vi "QT_QTImageToLVPict.vi"(1 "Draw info":bool, 2 "Image/Movie Out":T1={"Width"=160, "Height"=120, "Depth"=32, "data"=[], "Compressed data"=[], "Color table"=[], "Duration"=0, "Options"=0, "Timestamp"=0, "ID"=616, "Reserved"=0, "Dialogs"=0} {"Dialogs" format="%.0b"}, 3 "BW image":bool) -> (9 "Timestamp":i32, 13 "ID":i32=616, 14 "Picture color":picture, 16 "Picture B&W/Alpha channel":picture, 19 "Pict Draw Area Size":cluster{"Width":i16, "Height":i16}={"Width"=160, "Height"=120})   [LabVIEW 2024]
uses:
  <userlib>/ImageProcessing/QTLIB_2595_LV86/QT_Image.ctl
panel:
  in  "1 bit image":bool
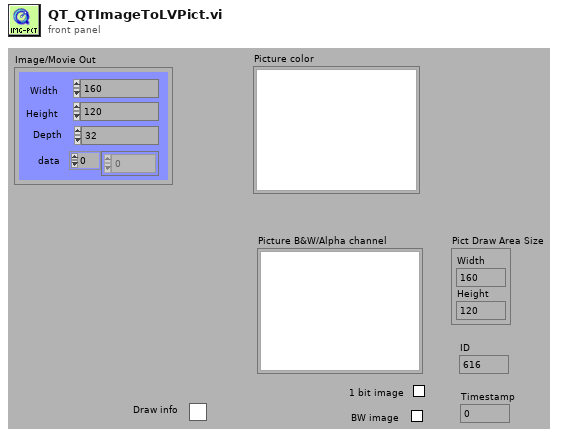
[diagram p1: front panel]
types:
  T1 = typedef "QT_Image.ctl" = cluster{"Width":i32, "Height":i32, "Depth":i32, "data":u8[], "Compressed data":u8[], "Color table":u32[], "Duration":i32, "Options":i32, "Timestamp":i32, "ID":i32, "Reserved":i32, "Dialogs":u32}
  T2 = cluster{"left":i16, "top":i16, "right":i16, "bottom":i16}
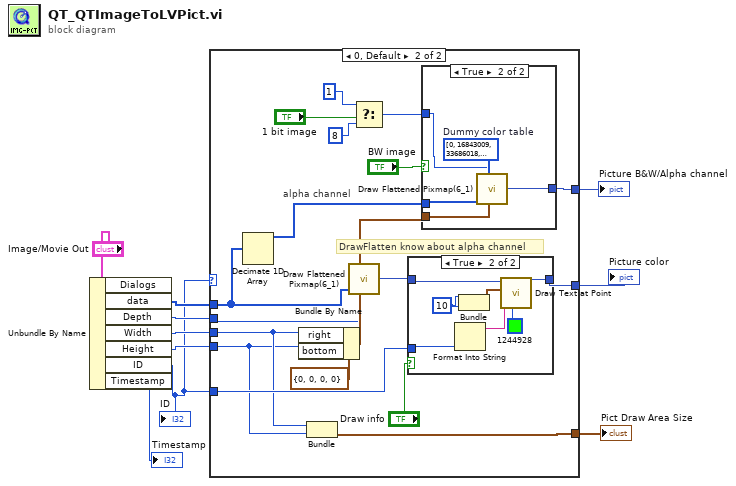
[diagram p0: block diagram]
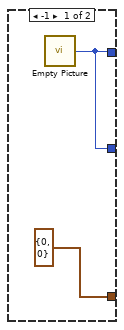
[diagram p2: hidden frame]
diagram:
  n1 = Unbundle By Name("Image/Movie Out") -> ("data"=w10:u8[], "Depth"=w8:i32, "Width"=w7:i32, "Height"=w6:i32, "ID"=w3:i32, "Timestamp"=→"Timestamp":i32)  [unwired: 1 out]
  "ID" <- w3
  n2 = case shown="0, Default" w3 {
    tunnel: w10 -> [_ w13]
    tunnel: w8 -> [_ w19]
    tunnel: w7 -> [_ w21]
    tunnel: w6 -> [_ w20]
    tunnel: [w12 w30] -> w5
    tunnel: [w12 w28] -> w4
    tunnel: w3 -> [_ w27]
    tunnel: [cluster{"Width":i16, "Height":i16} {"Width"=0, "Height"=0} ("Pict Draw Area Size") w22] -> w2
    frame -1 {
      n3 = call "Empty Picture"() -> ("empty picture"=w12:picture)
    }
    frame 0, Default {
      # "DrawFlatten know about alpha channel"
      # "alpha channel"
      n4 = Decimate 1D Array(w13) -> (w14:u8[])  [unwired: 3 out]
      n5 = Bundle By Name(cluster=T2 {"left"=0, "top"=0, "right"=0, "bottom"=0} ("rect"), "right"=w21, "bottom"=w20) -> (w23:T2)
      n6 = Bundle("Width"=w21, "Height"=w20) -> (w22:cluster{"Width":i32, "Height":i32})  [unwired: 1 out]
      n7 = call <vilib>:"Draw Flattened Pixmap(6_1).vi"("bit depth(8)"=w19, "rect"=w23, "flattened pixmap data"=w13) -> ("new picture"=w29:picture)  [unwired: 2 in, 4 out]
      n8 = Select(t=u8 1 ("bit depth(8)"), s="1 bit image", f=u8 8 ("bit depth(8)")) -> (s? t:f=w17:u8)
      n9 = case shown="True" "Draw info" {
        tunnel: w29 -> [w37 w44]
        tunnel: [w37 w43] -> w28
        tunnel: w27 -> [_ w39]
        frame False {
        }
        frame True {
          w40 = i16 10 ("left")
          n10 = Format Into String(w39) -> (resulting string=w38:string)  [unwired: 3 in, 1 out]
          n11 = Bundle("left"=w40, "left"=w40) -> (w42:cluster{"left":i16, "left":i16})  [unwired: 1 out]
          n12 = call <vilib>:"Draw Text at Point.vi"("text color(black)"=u32 1244928, "text"=w38, "origin"=w42, "picture"=w44) -> ("new picture"=w43:picture)  [unwired: 5 in, 2 out]
        }
      }
      n13 = case shown="True" "BW image" {
        tunnel: w14 -> [_ w36]
        tunnel: w23 -> [_ w35]
        tunnel: [w31 w34] -> w30
        tunnel: w17 -> [_ w32]
        frame False {
          n14 = call "Empty Picture"() -> ("empty picture"=w31:picture)
        }
        frame True {
          w33 = u32[] [0, 16843009, 33686018, 50529027, 67372036, 84215045, 101058054, 117901063, 134744072, 151587081, 168430090, 185273099, 202116108, 218959117, 235802126, 252645135, 269488144, 286331153, 303174162, 320017171, 336860180, 353703189, 370546198, 387389207, 404232216, 421075225, 437918234, 454761243, 471604252, 488447261, 505290270, 522133279, 538976288, 555819297, 572662306, 589505315, 606348324, 623191333, 640034342, 656877351, 673720360, 690563369, 707406378, 724249387, 741092396, 757935405, 774778414, 791621423, 808464432, 825307441, 842150450, 858993459, 875836468, 892679477, 909522486, 926365495, 943208504, 960051513, 976894522, 993737531, 1010580540, 1027423549, 1044266558, 1061109567, 1077952576, 1094795585, 1111638594, 1128481603, 1145324612, 1162167621, 1179010630, 1195853639, 1212696648, 1229539657, 1246382666, 1263225675, 1280068684, 1296911693, 1313754702, 1330597711, 1347440720, 1364283729, 1381126738, 1397969747, 1414812756, 1431655765, 1448498774, 1465341783, 1482184792, 1499027801, 1515870810, 1532713819, 1549556828, 1566399837, 1583242846, 1600085855, 1616928864, 1633771873, 1650614882, 1667457891, 1684300900, 1701143909, 1717986918, 1734829927, 1751672936, 1768515945, 1785358954, 1802201963, 1819044972, 1835887981, 1852730990, 1869573999, 1886417008, 1903260017, 1920103026, 1936946035, 1953789044, 1970632053, 1987475062, 2004318071, 2021161080, 2038004089, 2054847098, 2071690107, 2088533116, 2105376125, 2122219134, 2139062143, 2155905152, 2172748161, 2189591170, 2206434179, 2223277188, 2240120197, 2256963206, 2273806215, 2290649224, 2307492233, 2324335242, 2341178251, 2358021260, 2374864269, 2391707278, 2408550287, 2425393296, 2442236305, 2459079314, 2475922323, 2492765332, 2509608341, 2526451350, 2543294359, 2560137368, 2576980377, 2593823386, 2610666395, 2627509404, 2644352413, 2661195422, 2678038431, 2694881440, 2711724449, 2728567458, 2745410467, 2762253476, 2779096485, 2795939494, 2812782503, 2829625512, 2846468521, 2863311530, 2880154539, 2896997548, 2913840557, 2930683566, 2947526575, 2964369584, 2981212593, 2998055602, 3014898611, 3031741620, 3048584629, 3065427638, 3082270647, 3099113656, 3115956665, 3132799674, 3149642683, 3166485692, 3183328701, 3200171710, 3217014719, 3233857728, 3250700737, 3267543746, 3284386755, 3301229764, 3318072773, 3334915782, 3351758791, 3368601800, 3385444809, 3402287818, 3419130827, 3435973836, 3452816845, 3469659854, 3486502863, 3503345872, 3520188881, 3537031890, 3553874899, 3570717908, 3587560917, 3604403926, 3621246935, 3638089944, 3654932953, 3671775962, 3688618971, 3705461980, 3722304989, 3739147998, 3755991007, 3772834016, 3789677025, 3806520034, 3823363043, 3840206052, 3857049061, 3873892070, 3890735079, 3907578088, 3924421097, 3941264106, 3958107115, 3974950124, 3991793133, 4008636142, 4025479151, 4042322160, 4059165169, 4076008178, 4092851187, 4109694196, 4126537205, 4143380214, 4160223223, 4177066232, 4193909241, 4210752250, 4227595259, 4244438268, 4261281277, 4278124286, 4294967295]  # Dummy color table
          n15 = call <vilib>:"Draw Flattened Pixmap(6_1).vi"("bit depth(8)"=w32, "rect"=w35, "flattened pixmap data"=w36, "color table"=w33) -> ("new picture"=w34:picture)  [unwired: 1 in, 4 out]
        }
      }
    }
  }
  "Picture color" <- w4
  "Picture B&W/Alpha channel" <- w5
  "Pict Draw Area Size" <- w2
